vi "Setting_Screen_Enqueue Message.vi"   [LabVIEW 2024, in "Setting_Screen.lvlib" / "Setting_Screen_Message Queue.lvlib"]
doc: "For a regular message, enqueue the message. For a priority message, enqueue it at the front of the queue."
uses:
  Setting_Screen_Message Queue.lvlib
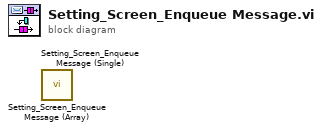
[diagram p0: block diagram]
diagram:
  n1 = call "Setting_Screen_Enqueue Message (Array).vi"() -> ()  [unwired: 10 in, 2 out]
  n2 = call "Setting_Screen_Enqueue Message (Single).vi"() -> ()  [unwired: 10 in, 2 out]
